vi "Close.vi"(8 "error in":errorcluster, 11 "VISA resource name":refnum<visa-resource-name>) -> (0 "error out":errorcluster)   [LabVIEW 2020, in "FirmataClient.lvlib"]
doc: "Closes the comport to the UUT / target"
uses:
  FirmataClient.lvlib
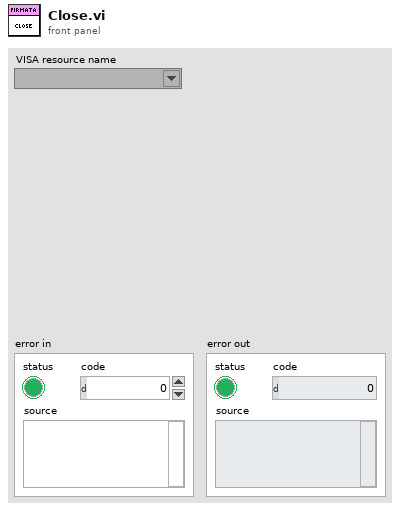
[diagram p1: front panel]
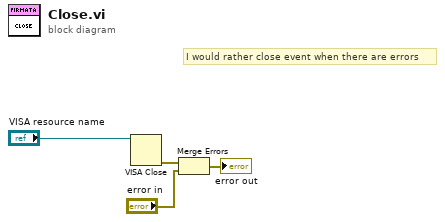
[diagram p0: block diagram]
diagram:
  # "I would rather close event when there are errors"
  n1 = VISA Close(VISA resource name="VISA resource name") -> (error out=w3:errorcluster)  [unwired: 1 in]
  n2 = Merge Errors(w3, "error in") -> (→"error out":errorcluster)
